vi "Finalize To Settings.vi"(8 "error in (no error)":errorcluster, 11 "UDP Rx Transfer Configuration in":refnum<class "UDP Transfer Rx Configuration.lvclass">) -> (0 "error out":errorcluster, 1 "settings version":T1, 2 "settings":cluster{"key":string, "value":string}[](array[cluster]), 3 "UDP Rx Transfer Configuration out":refnum<class "UDP Transfer Rx Configuration.lvclass">)   [LabVIEW 2017, in "DSF Core.lvlib" / "UDP Transfer Rx Configuration.lvclass"]
uses:
  UDP Transfer Rx Configuration.lvclass
  Typedefs/DSF Version Info.ctl
  UDP Transfer Rx Configuration.lvclass/UDP Transfer Rx Configuration.ctl
  DSF Core.lvlib
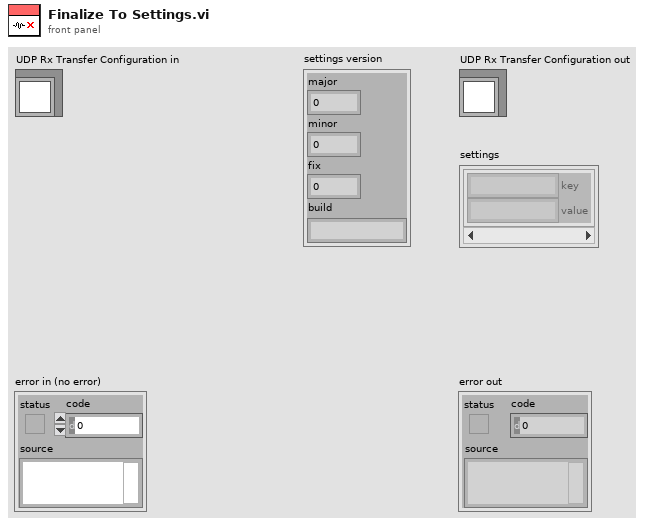
[diagram p1: front panel]
types:
  T1 = typedef "DSF Core.lvlib/DSF Version Info.ctl" = cluster{"major":u32, "minor":u32, "fix":u32, "build":string}
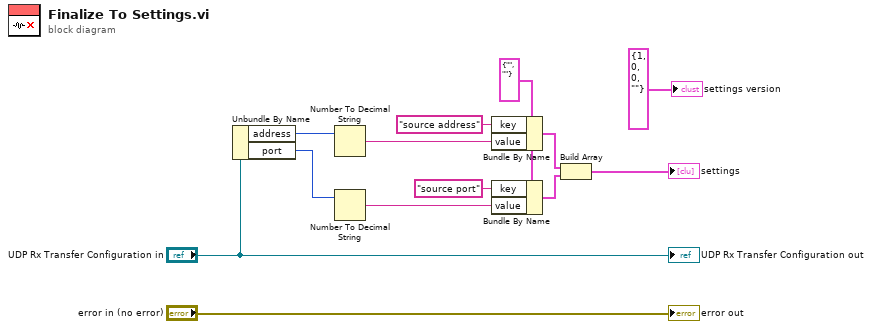
[diagram p0: block diagram]
diagram:
  w2 = cluster{"key":string, "value":string} {"key"="", "value"=""} ("setting")
  n1 = Unbundle By Name("UDP Rx Transfer Configuration in") -> ("address"=w7:u32, "port"=w6:u16)
  n2 = Number To Decimal String(number=w7) -> (decimal integer string=w13:string)  [unwired: 1 in]
  n3 = Number To Decimal String(number=w6) -> (decimal integer string=w8:string)  [unwired: 1 in]
  n4 = Bundle By Name(cluster=w2, "key"="source address", "value"=w13) -> (w9:cluster{"key":string, "value":string})
  n5 = Bundle By Name(cluster=w2, "key"="source port", "value"=w8) -> (w10:cluster{"key":string, "value":string})
  n6 = Build Array(w9, w10) -> (→"settings":cluster{"key":string, "value":string}[])
  "error out" <- "error in (no error)"
  "UDP Rx Transfer Configuration out" <- "UDP Rx Transfer Configuration in"
  "settings version" <- T1 {"major"=1, "minor"=0, "fix"=0, "build"=""} ("settings version")
